vi "angletoservo.vi"(8 "角度翻转":bool, 9 "手指":dbl, 10 "最小值":dbl, 11 "最大值输入":dbl) -> (3 "最大值输出":dbl)   [LabVIEW 2016]
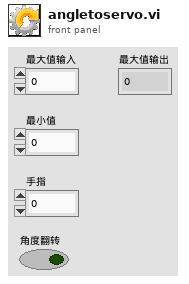
[diagram p1: front panel]
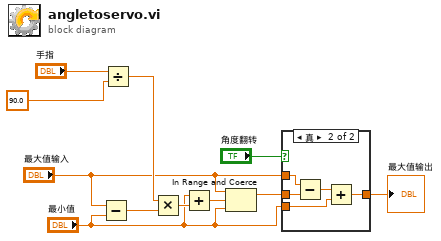
[diagram p0: block diagram]
diagram:
  n1 = Subtract(x="最大值输入", y="最小值") -> (x-y=w8:dbl)
  n2 = Divide(x="手指", y=90.0) -> (x/y=w7:dbl)
  n3 = Multiply(x=w7, y=w8) -> (x*y=w9:dbl)
  n4 = Add(x="最小值", y=w9) -> (x+y=w10:dbl)
  n5 = In Range and Coerce(upper limit="最大值输入", x=w10, lower limit="最小值") -> (coerced(x)=w4:dbl)  [unwired: 1 out]
  n6 = case shown="真" "角度翻转" {
    tunnel: w4 -> [w12 w16]
    tunnel: [w12 w13] -> w3
    tunnel: "最大值输入" -> [_ w17]
    tunnel: "最小值" -> [_ w14]
    frame False {
    }
    frame True {
      n7 = Subtract(x=w17, y=w16) -> (x-y=w15:dbl)
      n8 = Add(x=w15, y=w14) -> (x+y=w13:dbl)
    }
  }
  "最大值输出" <- w3
